vi "Get Column Template code.vi"   [LabVIEW 2023, in "SQLite.lvlib"]
doc: "Code template for extracting data from all returned rows."
uses:
  SQLite.lvlib
  SQL Statement.lvclass
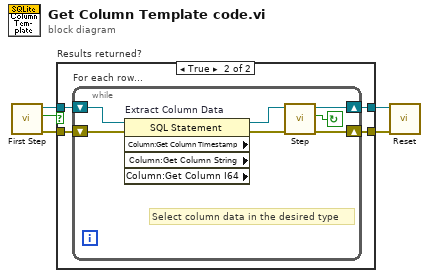
[diagram p0: block diagram]
diagram:
  n1 = call "First Step.vi"() -> ("error out"=w4:errorcluster, "Row returned"=w5:bool, "SQL Statement out"=w3:refnum<class "SQL Statement.lvclass">)  [unwired: 9 in]
  n2 = case "Results returned?" shown="True" w5 {
    tunnel: [w7 w11] -> w2
    tunnel: [w6 w10] -> w1
    tunnel: w3 -> [w7 w9]
    tunnel: w4 -> [w6 w8]
    frame False {
    }
    frame True {
      n3 = while "For each row..." {
        shift-right: [w17] -> w11
        shift-left: w9 -> [w14]
        shift-right: [w15] -> w10
        shift-left: w8 -> [w13]
        stop <- w12 continue-if-true
        # "Select column data in the desired type"
        n4 = property on="Extract Column Data" class="SQL Statement" props=["Column:Get Column Timestamp", "Column:Get Column String", "Column:Get Column I64"](reference=w14, error in=w13) -> (reference out=w18:refnum<class "SQL Statement.lvclass">, error out=w16:errorcluster)  [unwired: 3 out]
        n5 = call "Step.vi"("error in (no error)"=w16, "SQL Statement in"=w18) -> ("error out"=w15:errorcluster, "Row returned"=w12:bool, "SQL Statement out"=w17:refnum<class "SQL Statement.lvclass">)  [unwired: 7 in]
      }
    }
  }
  n6 = call "Reset.vi"("error in (no error)"=w1, "SQL Statement in"=w2) -> ()  [unwired: 8 in, 2 out]
